vi "startNewLog.vi"(8 "error in (no error)":errorcluster, 11 "Logger in":refnum<class "Log.lvclass">) -> (0 "error out":errorcluster, 3 "Logger out":refnum<class "Log.lvclass">)   [LabVIEW 2013, in "Log.lvlib" / "Log.lvclass"]
uses:
  <userlib>/Common/Log/Log/Log.lvclass
  <userlib>/Common/Log/Log/Log.lvclass/Log.ctl
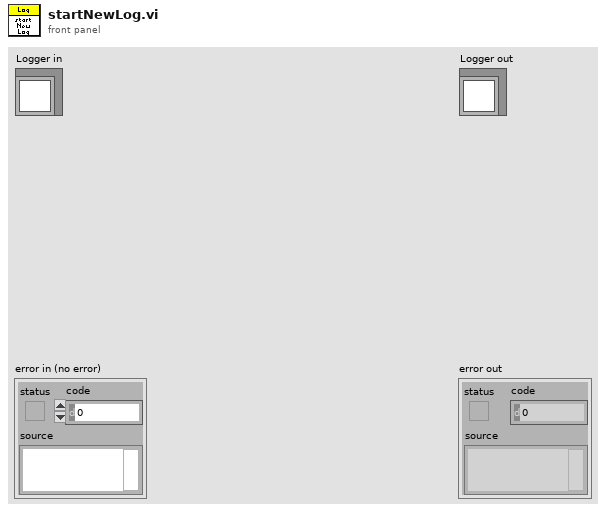
[diagram p1: front panel]
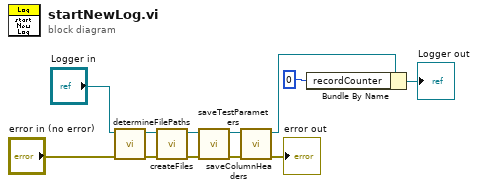
[diagram p0: block diagram]
diagram:
  n1 = call <userlib>:"determineFilePaths.vi"("error in (no error)"="error in (no error)", "Logger in"="Logger in") -> ("error out"=w2:errorcluster, "Logger out"=w4:refnum<class "Log.lvclass">)  [unwired: 8 in]
  n2 = call <userlib>:"createFiles.vi"("error in (no error)"=w2, "Log in"=w4) -> ("error out"=w1:errorcluster, "Log out"=w3:refnum<class "Log.lvclass">)  [unwired: 8 in]
  n3 = call-dynamic "saveTestParameters.vi"("error in (no error)"=w1, "Logger in"=w3) -> ("error out"=w7:errorcluster, "Logger out"=w8:refnum<class "Log.lvclass">)  [unwired: 8 in]
  n4 = call <userlib>:"saveColumnHeaders.vi"("error in (no error)"=w7, "Logger in"=w8) -> ("error out"=→"error out":errorcluster, "Logger out"=w11:refnum<class "Log.lvclass">)  [unwired: 8 in]
  n5 = Bundle By Name(cluster=w11, "recordCounter"=u32 0) -> (→"Logger out":refnum<class "Log.lvclass">)
